vi "KRASS Hiport_waiting time to read.vi"(8 "error in (no error)":errorcluster, 10 "spreadsheet string":string) -> (0 "error out":errorcluster, 2 "Numeric":dbl, 3 "CommandList":string[](array[string]))   [LabVIEW 2015]
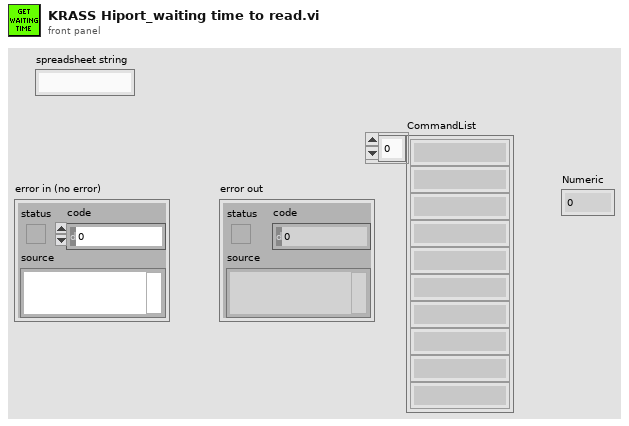
[diagram p1: front panel]
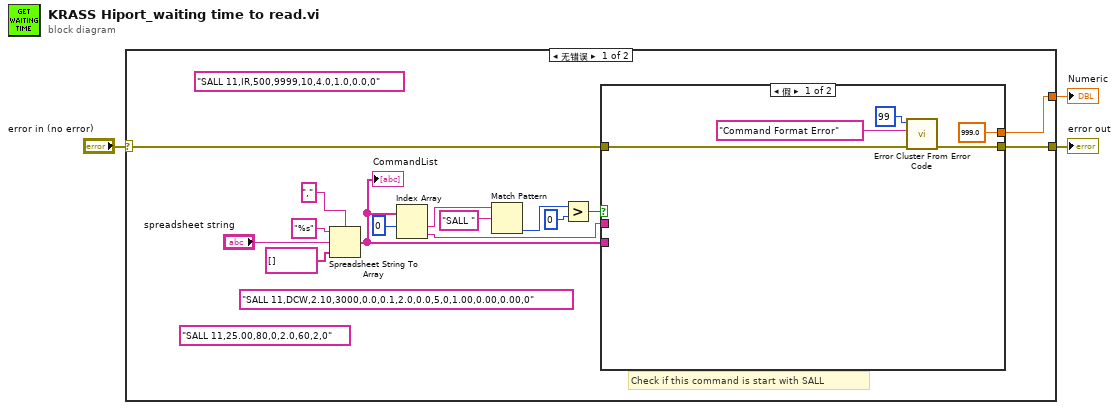
[diagram p0: block diagram]
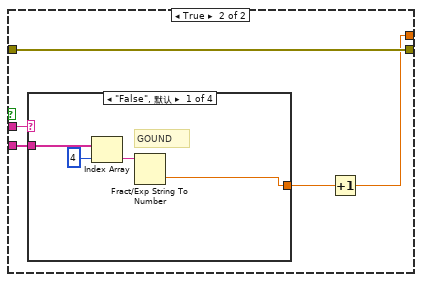
[diagram p2: hidden frame]
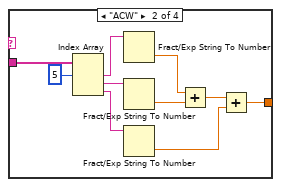
[diagram p3: hidden frame]
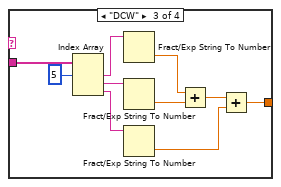
[diagram p4: hidden frame]
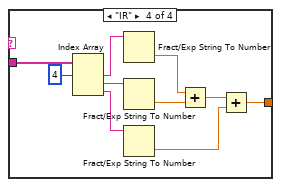
[diagram p5: hidden frame]
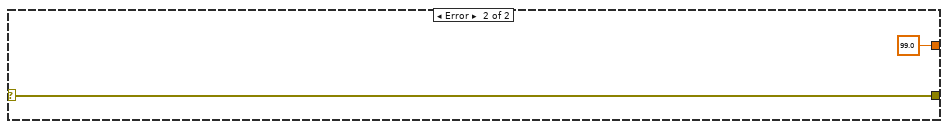
[diagram p6: hidden frame]
diagram:
  n1 = case shown="无错误" "error in (no error)" {
    selector: "error in (no error)" -> [w6 w63]
    tunnel: [w5 99.0] -> w1
    tunnel: [w4 w63] -> w2
    frame No Error {
      (unwired) "SALL 11,DCW,2.10,3000,0.0,0.1,2.0,0.0,5,0,1.00,0.00,0.00,0" ("write buffer")
      (unwired) "SALL 11,IR,500,9999,10,4.0,1.0,0.0,0" ("write buffer")
      (unwired) "SALL 11,25.00,80,0,2.0,60,2,0" ("write buffer")
      # "Check if this command is start with SALL"
      n2 = Spreadsheet String To Array(delimiter (Tab)=",", format string="%s", spreadsheet string="spreadsheet string", array type (2D Dbl)=string[] []) -> (array=w14:string[])
      "CommandList" <- w14
      n3 = Index Array(array=w14, index #1=0 ("index")) -> (element #1=w11:string, element #2=w12:string)  [unwired: 1 in]
      n4 = Match Pattern(string=w11, regular expression="SALL ") -> (offset past match=w9:i32)  [unwired: 1 in, 3 out]
      n5 = Greater?(x=w9, y=0) -> (0:w7:bool)
      n6 = case shown="假" w7 {
        tunnel: w14 -> [_ w28]
        tunnel: [999.0 w24] -> w5
        tunnel: w12 -> [_ w26]
        tunnel: w6 -> [w23 w25]
        tunnel: [w20 w25] -> w4
        frame False {
          n7 = call <vilib>:"Error Cluster From Error Code.vi"("error in (no error)"=w23, "error message (\"\")"="Command Format Error" ("error message (\"\")"), "error code (0)"=99) -> ("error out"=w20:errorcluster)  [unwired: 6 in]
        }
        frame True {
          n8 = case shown="\"False\", 默认" w26 {
            tunnel: w28 -> [w32 w35 w46 w56]
            tunnel: [w29 w34 w44 w54] -> w27
            frame "False", Default {
              # "GOUND"
              n9 = Index Array(array=w32, index=4) -> (element=w30:string)
              n10 = Fract/Exp String To Number(string=w30) -> (number=w29:dbl)  [unwired: 3 in, 1 out]
            }
            frame "ACW" {
              n11 = Index Array(array=w35, index #1=5 ("index")) -> (element #1=w41:string, element #2=w40:string, element #3=w33:string)  [unwired: 2 in]
              n12 = Fract/Exp String To Number(string=w41) -> (number=w39:dbl)  [unwired: 3 in, 1 out]
              n13 = Fract/Exp String To Number(string=w40) -> (number=w38:dbl)  [unwired: 3 in, 1 out]
              n14 = Fract/Exp String To Number(string=w33) -> (number=w36:dbl)  [unwired: 3 in, 1 out]
              n15 = Add(x=w39, y=w38) -> (x+y=w37:dbl)
              n16 = Add(x=w37, y=w36) -> (x+y=w34:dbl)
            }
            frame "DCW" {
              n17 = Index Array(array=w46, index #1=5 ("index")) -> (element #1=w51:string, element #2=w50:string, element #3=w43:string)  [unwired: 2 in]
              n18 = Fract/Exp String To Number(string=w51) -> (number=w49:dbl)  [unwired: 3 in, 1 out]
              n19 = Fract/Exp String To Number(string=w50) -> (number=w48:dbl)  [unwired: 3 in, 1 out]
              n20 = Fract/Exp String To Number(string=w43) -> (number=w45:dbl)  [unwired: 3 in, 1 out]
              n21 = Add(x=w49, y=w48) -> (x+y=w47:dbl)
              n22 = Add(x=w47, y=w45) -> (x+y=w44:dbl)
            }
            frame "IR" {
              n23 = Index Array(array=w56, index #1=4 ("index")) -> (element #1=w61:string, element #2=w60:string, element #3=w53:string)  [unwired: 2 in]
              n24 = Fract/Exp String To Number(string=w61) -> (number=w59:dbl)  [unwired: 3 in, 1 out]
              n25 = Fract/Exp String To Number(string=w60) -> (number=w58:dbl)  [unwired: 3 in, 1 out]
              n26 = Fract/Exp String To Number(string=w53) -> (number=w55:dbl)  [unwired: 3 in, 1 out]
              n27 = Add(x=w59, y=w58) -> (x+y=w57:dbl)
              n28 = Add(x=w57, y=w55) -> (x+y=w54:dbl)
            }
          }
          n29 = Increment(x=w27) -> (x+1=w24:dbl)
        }
      }
    }
    frame Error {
    }
  }
  "error out" <- w2
  "Numeric" <- w1
